vi "Open File on Disk.vi"(8 "error in":errorcluster, 11 "file or directory path":path) -> (0 "error out":errorcluster)   [LabVIEW 2019, in "Panther Dashboard.lvlib"]
uses:
  Panther Dashboard.lvlib
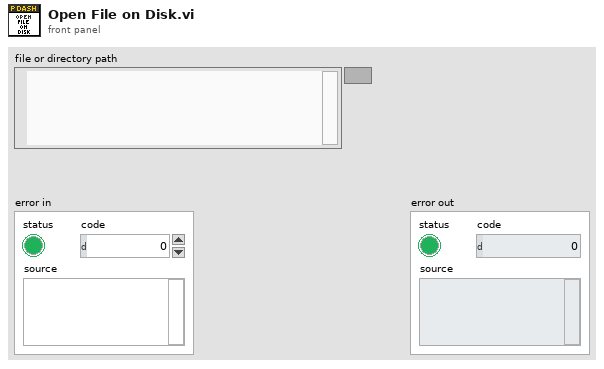
[diagram p1: front panel]
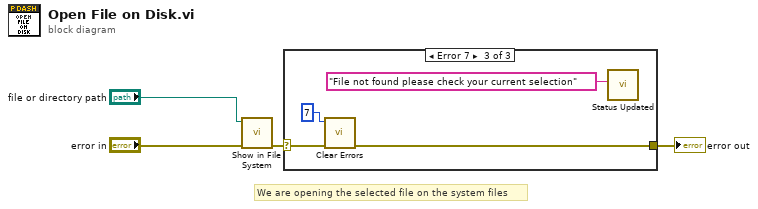
[diagram p0: block diagram]
diagram:
  # "We are opening the selected file on the system files"
  n1 = call <vilib>:"Show in File System.vi"("error in (no error)"="error in", "file or directory path"="file or directory path") -> ("error out"=w2:errorcluster)  [unwired: 9 in]
  n2 = case shown="Error 7" w2 {
    selector: w2 -> [w5 w6 w9]
    tunnel: [w5 w6 w10] -> w4
    frame No Error {
    }
    frame Default {
    }
    frame Error {
      n3 = call <vilib>:"Clear Errors.vi"("error in (no error)"=w9, "specific error code to clear (0: all)"=7) -> ("error out"=w10:errorcluster)  [unwired: 4 in, 1 out]
      n4 = call "Status Updated.vi"("Status"="File not found please check your current selection") -> ()  [unwired: 10 in, 1 out]
    }
  }
  "error out" <- w4
